vi "Update FIFO Full Flag - 16-bit Address.vi"(0 "full in":bool, 5 "full count in":u16, 7 "write":bool, 9 "read":bool, 11 "fifo depth":T1=10 items=["4"=2, "8"=3, "16"=4, "32"=5, "64"=6, "128"=7, "256"=8, "512"=9, "1024"=10, "2048"=11, "4096"=12, "8192"=13, "16384"=14, "32768"=15, "65536"=16]) -> (4 "full out":bool, 6 "full count out":u16)   [LabVIEW 2011, in "FIFO.lvlib"]
uses:
  <instrlib>/RF-RIO/FIFO/FIFO/FPGA/FIFO.lvlib
  <instrlib>/RF-RIO/FIFO/FIFO/FPGA/Private/FIFO Depth - 16-bit Address.ctl
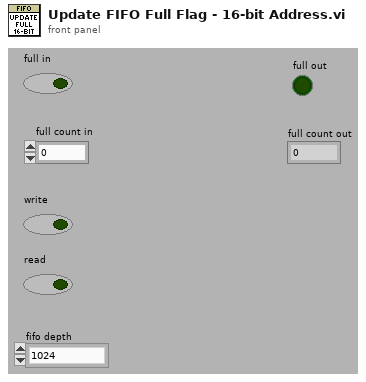
[diagram p1: front panel]
types:
  T1 = typedef "FIFO.lvlib/FIFO Depth - 16-bit Address.ctl" = u8
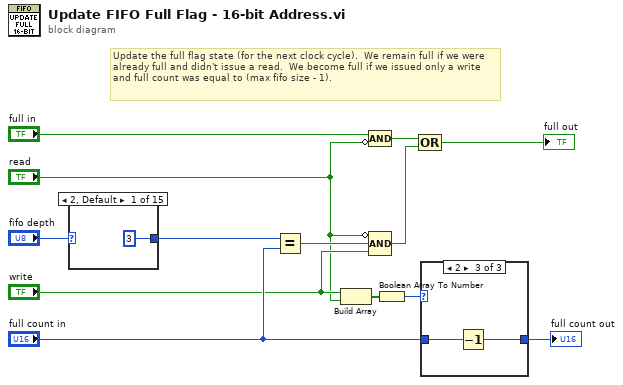
[diagram p0: block diagram]
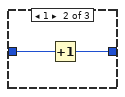
[diagram p3: hidden frame]
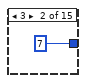
[diagram p4: hidden frame]
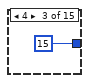
[diagram p5: hidden frame]
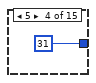
[diagram p6: hidden frame]
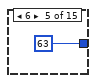
[diagram p7: hidden frame]
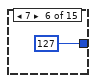
[diagram p8: hidden frame]
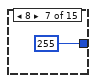
[diagram p9: hidden frame]
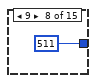
[diagram p10: hidden frame]
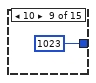
[diagram p11: hidden frame]
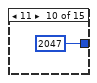
[diagram p12: hidden frame]
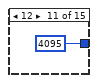
[diagram p13: hidden frame]
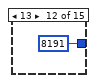
[diagram p14: hidden frame]
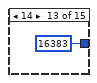
[diagram p15: hidden frame]
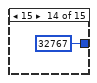
[diagram p16: hidden frame]
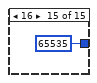
[diagram p17: hidden frame]
diagram:
  # "Update the full flag state (for the next clock cycle).  We remain full if we were already full and didn't issue a read.  We become full if we issued only a write and full count was equal to (max fifo size - 1)."
  n1 = case shown="2, Default" "fifo depth" {
    tunnel: [u16 3 u16 7 u16 15 u16 31 u16 63 u16 127 u16 255 u16 511 u16 1023 u16 2047 u16 4095 u16 8191 u16 16383 u16 32767 u16 65535] -> w7
    frame 2, Default {
    }
    frame 3 {
    }
    frame 4 {
    }
    frame 5 {
    }
    frame 6 {
    }
    frame 7 {
    }
    frame 8 {
    }
    frame 9 {
    }
    frame 10 {
    }
    frame 11 {
    }
    frame 12 {
    }
    frame 13 {
    }
    frame 14 {
    }
    frame 15 {
    }
    frame 16 {
    }
  }
  n2 = Equal?(x=w7, y="full count in") -> (x = y?=w13:bool)
  n3 = Build Array("write", "read") -> (w6:bool[])
  n4 = Compound Arithmetic op=AND("full in", invert "read") -> (w12:bool)
  n5 = Compound Arithmetic op=AND(invert "read", w13, "write") -> (w11:bool)
  n6 = Boolean Array To Number(Boolean array=w6) -> (number=w5:u8)
  n7 = Compound Arithmetic op=OR(w12, w11) -> (→"full out":bool)
  n8 = case shown="2" w5 {
    tunnel: "full count in" -> [w29 w31 w33]
    tunnel: [w29 w30 w32] -> w4
    frame 0, 3, Default {
    }
    frame 1 {
      n9 = Increment(x=w31) -> (x+1=w30:u16)
    }
    frame 2 {
      n10 = Decrement(x=w33) -> (x-1=w32:u16)
    }
  }
  "full count out" <- w4
